vi "Close.vi"(8 "error in (no error)":errorcluster, 11 "Chroma 19020":refnum<class "Chroma 190020.lvclass">) -> (0 "error out":errorcluster, 3 "Chroma 19020 out":refnum<class "Chroma 190020.lvclass">)   [LabVIEW 2025, in "HiPOT.lvlib" / "Chroma 190020.lvclass"]
uses:
  Chroma 190020.lvclass
  Chroma 190020.lvclass/Chroma 190020.ctl
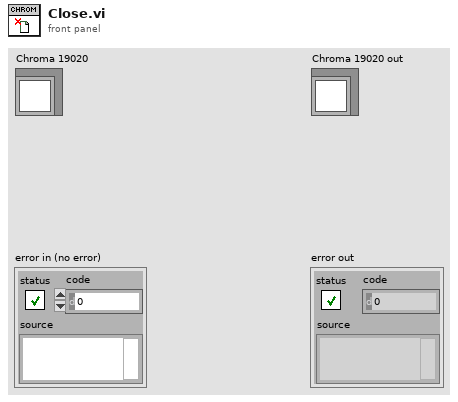
[diagram p1: front panel]
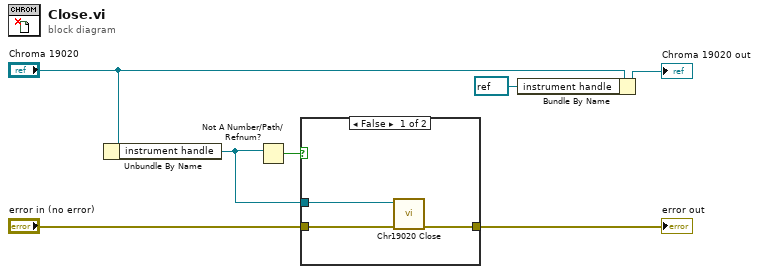
[diagram p0: block diagram]
diagram:
  n1 = Unbundle By Name("Chroma 19020") -> ("instrument handle"=w6:refnum<k15>)
  n2 = Not A Number/Path/Refnum?(number/path/refnum=w6) -> (NaN/Path/Refnum?=w7:bool)
  n3 = case shown="False" w7 {
    tunnel: [w9 w11] -> w2
    tunnel: "error in (no error)" -> [w10 w11]
    tunnel: w6 -> [w8 _]
    frame False {
      n4 = call <instrlib>:"Chr19020 Close.vi"("error in (no error)"=w10, "instrument handle"=w8) -> ("error out"=w9:errorcluster)  [unwired: 9 in]
    }
    frame True {
    }
  }
  "error out" <- w2
  n5 = Bundle By Name(cluster="Chroma 19020", "instrument handle"=refnum<k15> refnum) -> (→"Chroma 19020 out":refnum<class "Chroma 190020.lvclass">)
